vi "LWXPS_GroupJogCurrentGet.vi"(0 "XPS Reference IN":refnum<k24>, 1 "Group Name":string, 2 "Number of positioners":i32, 5 "LabVIEW error IN":errorcluster) -> (14 "XPS Reference OUT":refnum<k24>, 15 "Returned error code":i32, 16 "Velocity":dbl[](array[numeric]), 17 "Acceleration":dbl[](array[numeric]), 18 "XPS Error String":string, 19 "LabVIEW error OUT":errorcluster)   [LabVIEW 2014]
uses:
  D:/XPSQ8_LabView_Library/Development/Source/Dll/Newport.XPS.CommandInterface.dll
  Dll/Newport.XPS.CommandInterface.dll
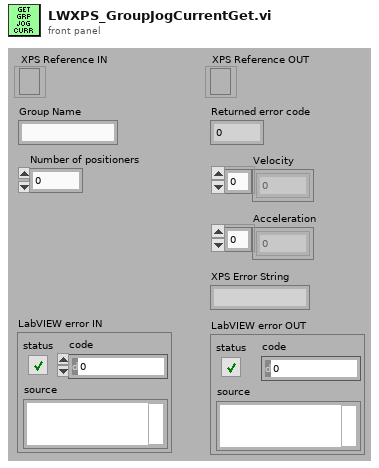
[diagram p1: front panel]
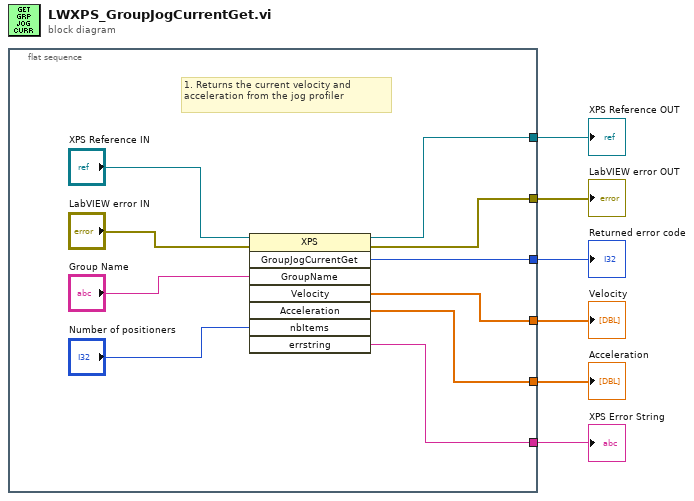
[diagram p0: block diagram]
diagram:
  n1 = flat-sequence {
    tunnel: [w8] -> w6
    tunnel: [w13] -> w5
    tunnel: [w15] -> w4
    tunnel: [w12] -> w2
    tunnel: [w7] -> w1
    tunnel: [w9] -> w3
    frame #0 {
      # "1. Returns the current velocity and acceleration from the jog profiler"
      n2 = invoke class="XPS" method="GroupJogCurrentGet"(reference="XPS Reference IN", error in="LabVIEW error IN", "GroupName"="Group Name", "nbItems"="Number of positioners") -> (reference out=w8:refnum<k24>, error out=w13:errorcluster, "GroupJogCurrentGet"=w15:i32, "Velocity"=w9:dbl[], "Acceleration"=w12:dbl[], "errstring"=w7:string)  [unwired: 4 in, 2 out]
    }
  }
  "XPS Reference OUT" <- w6
  "LabVIEW error OUT" <- w5
  "Returned error code" <- w4
  "XPS Error String" <- w1
  "Velocity" <- w3
  "Acceleration" <- w2
